vi "ReadPersonnel.vi"(8 "error in (no error)":errorcluster, 11 "PUID":string) -> (0 "error out":errorcluster, 2 "Personnel":string)   [LabVIEW 2015, in "PersonnelRestApi.lvlib"]
uses:
  PersonnelRestApi.lvlib
  TypeDef/GetPersonnelCommands.ctl
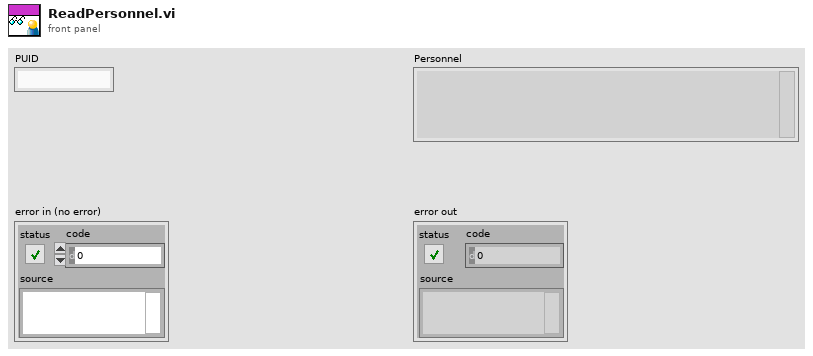
[diagram p1: front panel]
types:
  T1 = typedef "PersonnelRestApi.lvlib/GetPersonnelCommands.ctl" = enum16{"ReadPersonnel", "ReadName", "ReadRole", "ReadRequests", "ReadPUIDs"}
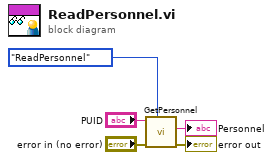
[diagram p0: block diagram]
diagram:
  n1 = call "GetPersonnel.vi"("Room Commands"=GetPersonnelCommands."ReadPersonnel", "error in (no error)"="error in (no error)", "PUID"="PUID") -> ("error out"=→"error out":errorcluster, "JSON"=→"Personnel":string)  [unwired: 7 in]
